vi "Save_Raw_data.vi"(6 "Meas_rang":i32[](array[numeric]), 8 "错误输入（无错误）":errorcluster, 9 "Data_struct":refnum<k24>[](array[refnum]), 10 "Meas_monitor_struct":refnum<k24>[](array[refnum]), 11 "ILSTS":refnum<k24>) -> (0 "错误输出":errorcluster)   [LabVIEW 2017]
doc: "Save mesurement raw data"
uses:
  D:/test/ILSTS/LV_IL/LV_IL_Sample_x86/DLL/STSProcess.dll
  DLL/STSProcess.dll
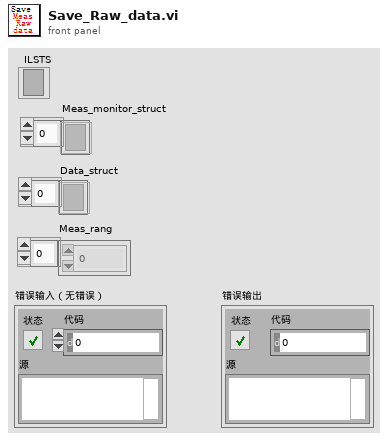
[diagram p1: front panel]
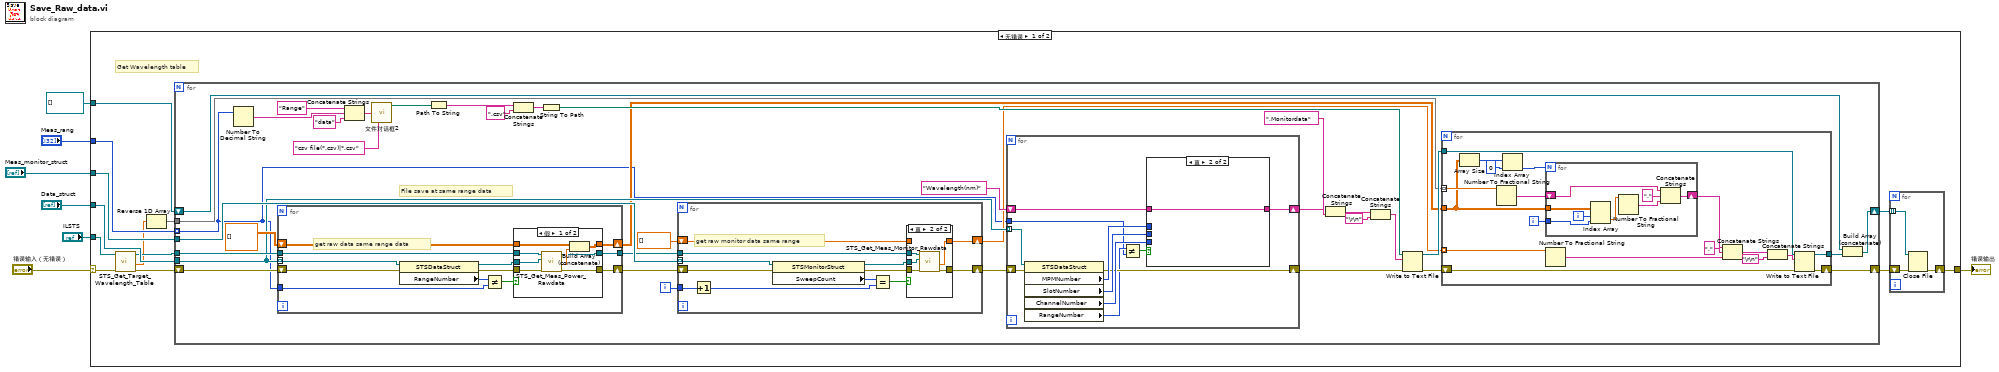
[diagram p0: block diagram]
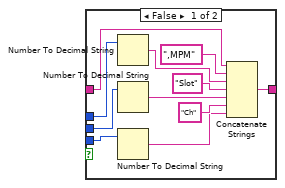
[diagram p2: hidden frame]
diagram:
  n1 = case shown="无错误" "错误输入（无错误）" {
    selector: "错误输入（无错误）" -> [w19 w152]
    tunnel: [w12 w152] -> w7
    tunnel: "ILSTS" -> [w20 _]
    tunnel: "Data_struct" -> [w17 _]
    tunnel: "Meas_rang" -> [w18 _]
    tunnel: "Meas_monitor_struct" -> [w16 _]
    tunnel: refnum<file>[] [] ("添加的数组") -> [w15 _]
    frame No Error {
      # "Get Wavelength table"
      n2 = call "STS_Get_Target_Wavelength_Table.vi"("错误输入（无错误）"=w19, ".NET引用句柄输入"=w20) -> ("error out"=w11:errorcluster, "wavelengths"=w9:dbl[], "引用输出"=w10:refnum<k24>)  [unwired: 7 in]
      n3 = Reverse 1D Array(array=w9) -> (reversed array=w8:dbl[])
      n4 = for {
        tunnel: w17 -> [w41]
        tunnel: w18 -> [w21] mode=indexing
        tunnel: w10 -> [w56]
        shift-right: [w24] -> w13
        shift-left: w11 -> [w57]
        tunnel: w16 -> [w55]
        tunnel: w8 -> [w30]
        shift-right: [w26] -> w14
        shift-left: w15 -> [w25]
        i -> [w22]
        # "File save at same range data"
        n5 = Number To Decimal String(number=w21) -> (decimal integer string=w51:string)  [unwired: 1 in]
        n6 = for {
          tunnel: w41 -> [w137] mode=indexing
          tunnel: w21 -> [w135]
          tunnel: w56 -> [w131]
          shift-right: [w127] -> w54
          shift-left: w57 -> [w133]
          shift-right: [w128] -> w28
          shift-left: sgl[][] [] -> [w129]
          tunnel: [w126] -> w53
          # "get raw data same range data"
          n7 = property on="属性节点" class="STSDataStruct"(reference=w137, error in=w133) -> (reference out=w130:refnum<k24>, error out=w132:errorcluster, "RangeNumber"=w136:i32)
          n8 = Not Equal?(x=w136, y=w135) -> (x != y?=w134:bool)
          n9 = case shown="假" w134 {
            tunnel: w132 -> [w145 w147]
            tunnel: w131 -> [w144 w146]
            tunnel: w130 -> [w143 _]
            tunnel: w129 -> [w141 w148]
            tunnel: [w140 w148] -> w128
            tunnel: [w139 w147] -> w127
            tunnel: [w138 w146] -> w126
            frame False {
              n10 = call "STS_Get_Meas_Power_Rawdata.vi"("错误输入（无错误）"=w145, "setting"=w143, ".NET引用句柄输入"=w144) -> ("error out"=w139:errorcluster, "powerdata"=w142:sgl[], "引用输出"=w138:refnum<k24>)  [unwired: 6 in]
              n11 = Build Array (concatenate)(w141, w142) -> (w140:sgl[][])
            }
            frame True {
            }
          }
        }
        n12 = Concatenate Strings("Range" ("字符串"), w51, "data" ("字符串")) -> (w47:string)
        n13 = call "文件对话框2"("default name"=w47, "pattern (all files)"="csv file(*.csv)|*.csv") -> ("selected path"=w43:path)  [unwired: 10 in, 3 out]
        n14 = Path To String(path=w43) -> (string=w44:string)
        n15 = Concatenate Strings(w44, ".csv" ("名称或相对路径")) -> (w45:string)
        n16 = String To Path(string=w45) -> (path=w35:path)
        n17 = for {
          tunnel: w55 -> [w118] mode=indexing
          shift-right: [w109] -> w33
          shift-left: w54 -> [w117]
          tunnel: w22 -> [w116]
          tunnel: w53 -> [w110]
          shift-right: [w108] -> w27
          shift-left: sgl[] [] ("monitordata") -> [w107]
          # "get raw monitor data same range"
          n18 = Increment(x=w116) -> (x+1=w114:i32)
          n19 = property on="属性节点" class="STSMonitorStruct"(reference=w118, error in=w117) -> (reference out=w112:refnum<k24>, error out=w111:errorcluster, "SweepCount"=w115:i32)
          n20 = Equal?(x=w115, y=w114) -> (x = y?=w113:bool)
          n21 = case shown="真" w113 {
            tunnel: w112 -> [_ w125]
            tunnel: w111 -> [w120 w124]
            tunnel: w110 -> [_ w123]
            tunnel: [w120 w122] -> w109
            tunnel: [w119 w121] -> w108
            tunnel: w107 -> [w119 _]
            frame False {
            }
            frame True {
              n22 = call "STS_Get_Meas_Monitor_Rawdata.vi"("错误输入（无错误）"=w124, "setting"=w125, ".NET引用句柄输入"=w123) -> ("error out"=w122:errorcluster, "monitordata"=w121:sgl[])  [unwired: 6 in, 1 out]
            }
          }
        }
        n23 = for {
          tunnel: w41 -> [w94] mode=indexing
          shift-right: [w88] -> w39
          shift-left: "Wavelength(nm)" -> [w89]
          shift-right: [w87] -> w34
          shift-left: w33 -> [w93]
          tunnel: w21 -> [w85]
          n24 = property on="属性节点" class="STSDataStruct"(reference=w94, error in=w93) -> (error out=w87:errorcluster, "MPMNumber"=w90:i32, "SlotNumber"=w91:i32, "ChannelNumber"=w92:i32, "RangeNumber"=w86:i32)  [unwired: 1 out]
          n25 = Not Equal?(x=w86, y=w85) -> (x != y?=w84:bool)
          n26 = case shown="真" w84 {
            tunnel: w92 -> [w105 _]
            tunnel: w91 -> [w104 _]
            tunnel: w90 -> [w103 _]
            tunnel: w89 -> [w102 w106]
            tunnel: [w95 w106] -> w88
            frame False {
              n27 = Number To Decimal String(number=w103) -> (decimal integer string=w100:string)  [unwired: 1 in]
              n28 = Number To Decimal String(number=w104) -> (decimal integer string=w98:string)  [unwired: 1 in]
              n29 = Number To Decimal String(number=w105) -> (decimal integer string=w96:string)  [unwired: 1 in]
              n30 = Concatenate Strings(w102, ",MPM" ("字符串"), w100, "Slot" ("字符串"), w98, "Ch" ("字符串"), w96) -> (w95:string)
            }
            frame True {
            }
          }
        }
        n31 = Concatenate Strings(w39, ",Monitordata" ("字符串")) -> (w36:string)
        n32 = Concatenate Strings(w36, "\r\n") -> (w38:string)
        n33 = Write to Text File(file (use dialog)=w35, text=w38, error in=w34) -> (refnum out=w31:refnum<file>, error out=w32:errorcluster)  [unwired: 1 in, 1 out]
        n34 = for {
          tunnel: w30 -> [w75] mode=indexing
          tunnel: w31 -> [w67]
          tunnel: [w66] -> w23
          shift-right: [w72] -> w24
          shift-left: w32 -> [w73]
          tunnel: w28 -> [w63]
          tunnel: w27 -> [w62] mode=indexing
          i -> [w64]
          n35 = Array Size(array=w63) -> (size(s)=w70:i32[])
          n36 = Number To Fractional String(number=w75) -> (F-format string=w74:string)  [unwired: 3 in]
          n37 = Index Array(array=w70, index=0 ("索引")) -> (element=w68:i32)
          n38 = for {
            N: w68 -> [_]
            tunnel: w63 -> [w83]
            tunnel: w64 -> [w82]
            shift-right: [w78] -> w59
            shift-left: w74 -> [w79]
            i -> [w81]
            n39 = Index Array(array=w83, index (row)=w81, index (col)=w82) -> (element=w80:sgl)
            n40 = Number To Fractional String(number=w80) -> (F-format string=w76:string)  [unwired: 3 in]
            n41 = Concatenate Strings(w79, "," ("字符串"), w76) -> (w78:string)
          }
          n42 = Number To Fractional String(number=w62) -> (F-format string=w61:string)  [unwired: 3 in]
          n43 = Concatenate Strings(w59, "," ("字符串"), w61) -> (w58:string)
          n44 = Concatenate Strings(w58, "\r\n") -> (w71:string)
          n45 = Write to Text File(file (use dialog)=w67, text=w71, error in=w73) -> (refnum out=w66:refnum<file>, error out=w72:errorcluster)  [unwired: 1 in, 1 out]
        }
        n46 = Build Array (concatenate)(w25, w23) -> (w26:refnum<file>[])
      }
      n47 = for {
        tunnel: w14 -> [w151] mode=indexing
        shift-right: [w149] -> w12
        shift-left: w13 -> [w150]
        n48 = Close File(refnum=w151, error in=w150) -> (error out=w149:errorcluster)  [unwired: 1 out]
      }
    }
    frame Error {
    }
  }
  "错误输出" <- w7
